vi "test_SomeSessRegistered_InitAndCloseSessWithAuto_InitAndCloseCalledWithProperBehavior.vi"(11 "error in":errorcluster) -> (4 "pass":bool, 6 "result":string, 15 "error out":errorcluster)   [LabVIEW 2020, in "MeasurementServerTests.lvlib"]
uses:
  MeasurementServerTests.lvlib
  Runtime/Clients/Session Management V1/Session Reservation/Initialize and Close Session Behavior.ctl
  Runtime/Clients/Session Management V1/Session Reservation/Session Reservation.lvclass
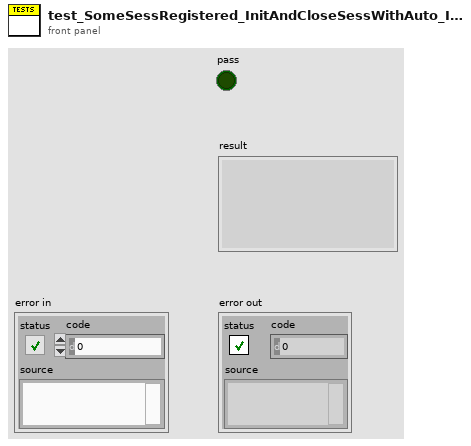
[diagram p1: front panel]
types:
  T1 = typedef "NI Session Management V1 Client.lvlib/Session Reservation.lvclass/Initialize and Close Session Behavior.ctl" = enum16{"Auto", "Initialize and Close", "Attach and Detach", "Initialize and Detach", "Attach and Close"}
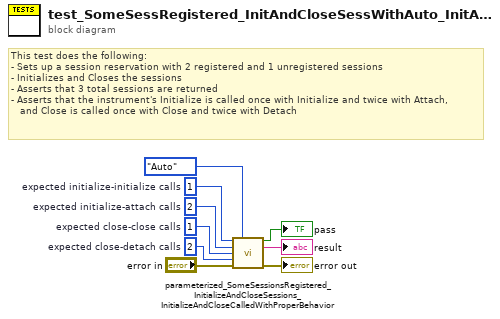
[diagram p0: block diagram]
diagram:
  w5 = u32 2  # expected close-detach calls
  w6 = u32 1  # expected close-close calls
  w7 = u32 2  # expected initialize-attach calls
  w8 = u32 1  # expected initialize-initialize calls
  # "This test does the following:\n- Sets up a session reservation with 2 registered and 1 unregistered sessions\n- Initializes and Closes the sessions\n- Asserts that 3 total sessions are returned\n- Asserts that the instrument's Initialize is called once with Initialize and twice with Attach,\n   and Close is called once with Close and twice with Detach"
  n1 = call "parameterized_SomeSessionsRegistered_InitializeAndCloseSessions_InitializeAndCloseCalledWithProperBehavior.vi"("expected initialize-initialize calls"=w8, "initialize and close session behavior"=Initialize_and_Close_Session_Behavior."Auto", "expected initialize-attach calls"=w7, "expected close-close calls"=w6, "expected close-detach calls"=w5, "error in"="error in") -> ("pass"=→"pass":bool, "result"=→"result":string, "error out"=→"error out":errorcluster)  [unwired: 7 in]
